vi "Acquire MultiSourceFrames.vi"() -> ()   [LabVIEW 2014]
uses:
  Microsoft.Kinect
panel:
  out "frameData":u8[](array[numeric])
  in  "stop":bool
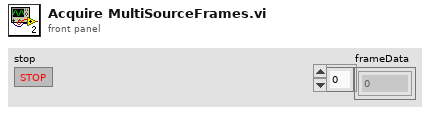
[diagram p1: front panel]
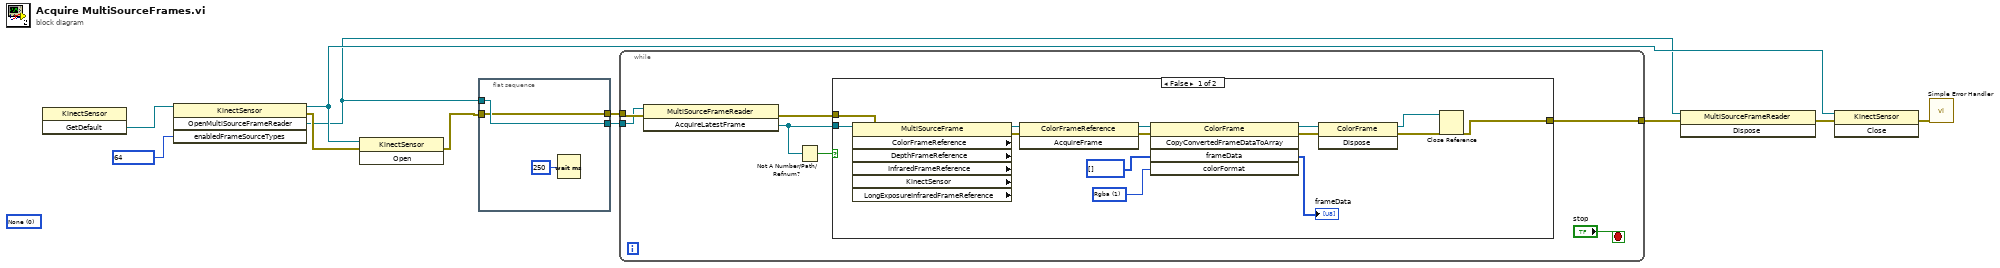
[diagram p0: block diagram]
diagram:
  (unwired) 0 items=["None"=0, "Color"=1, "Infrared"=2, "LongExposureInfrared"=4, "Depth"=8, "BodyIndex"=16, "Body"=32, "Audio"=64] ("enabledFrameSourceTypes")
  n1 = invoke class="KinectSensor" method="GetDefault"() -> ("GetDefault"=w11:refnum<k24>)  [unwired: 3 in, 2 out]
  n2 = invoke class="KinectSensor" method="OpenMultiSourceFrameReader"(reference=w11, "enabledFrameSourceTypes"=64) -> (reference out=w8:refnum<k24>, error out=w7:errorcluster, "OpenMultiSourceFrameReader"=w4:refnum<k24>)  [unwired: 2 in, 1 out]
  n3 = invoke class="KinectSensor" method="Open"(reference=w8, error in=w7) -> (error out=w5:errorcluster)  [unwired: 1 in, 2 out]
  n4 = flat-sequence {
    tunnel: w5 -> [w13]
    tunnel: w4 -> [w14]
    tunnel: [w14] -> w3
    tunnel: [w13] -> w2
    frame #0 {
      n5 = Wait (ms)(milliseconds to wait=u32 250) -> ()  [unwired: 1 out]
    }
  }
  n6 = while {
    tunnel: w2 -> [w21]
    tunnel: w3 -> [w15]
    tunnel: [w19] -> w6
    stop <- "stop" stop-if-true
    n7 = invoke class="MultiSourceFrameReader" method="AcquireLatestFrame"(reference=w15, error in=w21) -> (error out=w16:errorcluster, "AcquireLatestFrame"=w17:refnum<k24>)  [unwired: 1 in, 1 out]
    n8 = Not A Number/Path/Refnum?(number/path/refnum=w17) -> (NaN/Path/Refnum?=w18:bool)
    n9 = case shown="False" w18 {
      tunnel: w17 -> [w27 _]
      tunnel: [w22 w36] -> w19
      tunnel: w16 -> [w31 w36]
      frame False {
        w34 = 1 items=["None", "Rgba", "Yuv", "Bgra", "Bayer", "Yuy2"] ("colorFormat")
        n10 = property class="MultiSourceFrame" props=["ColorFrameReference", "DepthFrameReference", "InfraredFrameReference", "KinectSensor", "LongExposureInfraredFrameReference"](reference=w27, error in=w31) -> (error out=w30:errorcluster, "ColorFrameReference"=w26:refnum<k24>)  [unwired: 5 out]
        n11 = invoke class="ColorFrameReference" method="AcquireFrame"(reference=w26, error in=w30) -> (error out=w29:errorcluster, "AcquireFrame"=w35:refnum<k24>)  [unwired: 1 in, 1 out]
        n12 = invoke class="ColorFrame" method="CopyConvertedFrameDataToArray"(reference=w35, error in=w29, "frameData"=u8[] [], "colorFormat"=w34) -> (reference out=w32:refnum<k24>, error out=w28:errorcluster, "frameData"=→"frameData":u8[])  [unwired: 1 in, 2 out]
        n13 = invoke class="ColorFrame" method="Dispose"(reference=w32, error in=w28) -> (reference out=w23:refnum<k24>, error out=w24:errorcluster)  [unwired: 1 in, 1 out]
        n14 = Close Reference(reference=w23, error in (no error)=w24) -> (error out=w22:errorcluster)
      }
      frame True {
      }
    }
  }
  n15 = invoke class="MultiSourceFrameReader" method="Dispose"(reference=w4, error in=w6) -> (error out=w10:errorcluster)  [unwired: 1 in, 2 out]
  n16 = invoke class="KinectSensor" method="Close"(reference=w8, error in=w10) -> (error out=w9:errorcluster)  [unwired: 1 in, 2 out]
  n17 = call <vilib>:"Simple Error Handler.vi"("error in (no error)"=w9) -> ()  [unwired: 4 in, 5 out]
